vi "SUB instantant_frequency.vi"(2 "trimmed percent":cluster{"upper":dbl, "lower":dbl} {"lower" min=0.0 max=100.0 format="%#_g %"; "upper" min=0.0 max=100.0 format="%#_g %"}, 3 "scale info":variant, 4 "Omega":cluster{"frequency":dbl, "+- f":dbl}={"frequency"=444.0, "+- f"=50.0}, 5 "scalogram matrix":dbl[][](array[numeric])) -> (0 "IBandwidth":waveform(dbl), 1 "InstFrequency":waveform(dbl))   [LabVIEW 2017]
uses:
  <vilib>/addons/_Advanced Signal Processing/NI_AdvSigProcTFA.lvlib
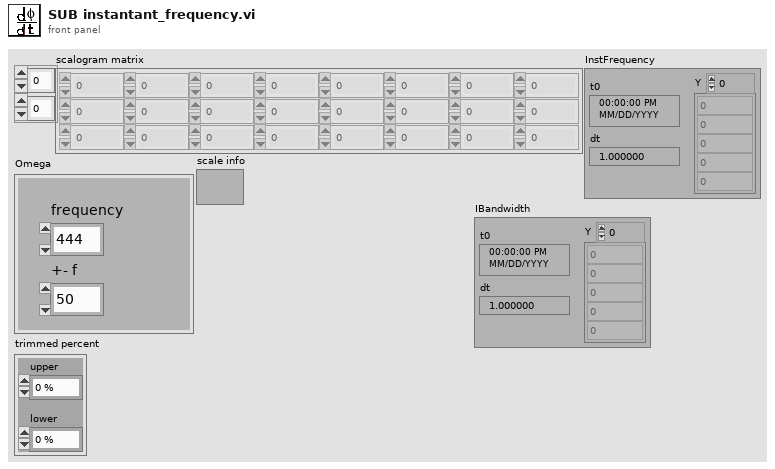
[diagram p1: front panel]
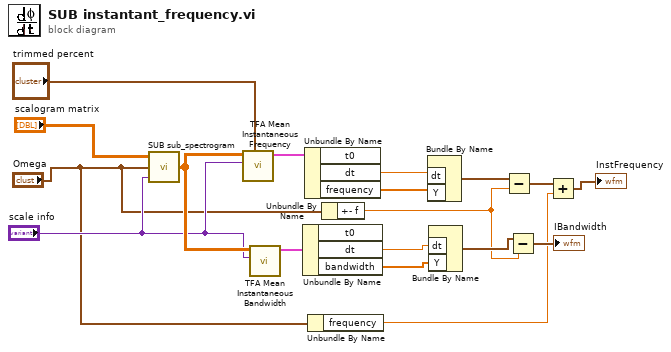
[diagram p0: block diagram]
diagram:
  n1 = call "SUB sub_spectrogram.vi"("scale info"="scale info", "Bandwidth"="Omega", "scalogram matrix"="scalogram matrix") -> ("sub_Spectrogram"=w14:cdb[][])
  n2 = call <vilib>:"TFA Mean Instantaneous Frequency.vi"("trimmed percent"="trimmed percent", "scale info"="scale info", "spectrogram"=w14) -> ("MIF"=w18:cluster{"t0":dbl, "dt":dbl, "frequency":dbl[]})  [unwired: 7 in, 1 out]
  n3 = call <vilib>:"TFA Mean Instantaneous Bandwidth.vi"("scale info"="scale info", "spectrogram"=w14) -> ("MIB"=w12:cluster{"t0":dbl, "dt":dbl, "bandwidth":dbl[]})  [unwired: 8 in, 1 out]
  n4 = Unbundle By Name(w12) -> ("dt"=w10:dbl, "bandwidth"=w9:dbl[])  [unwired: 1 out]
  n5 = Unbundle By Name(w18) -> ("dt"=w17:dbl, "frequency"=w16:dbl[])  [unwired: 1 out]
  n6 = Unbundle By Name("Omega") -> ("frequency"=w1:dbl)
  n7 = Unbundle By Name("Omega") -> ("+- f"=w7:dbl)
  n8 = Bundle By Name("dt"=w17, "Y"=w16) -> (w11:waveform(dbl))  [unwired: 1 in]
  n9 = Bundle By Name("dt"=w10, "Y"=w9) -> (w8:waveform(dbl))  [unwired: 1 in]
  n10 = Subtract(x=w11, y=w7) -> (x-y=w3:waveform(dbl))
  n11 = Subtract(x=w8, y=w7) -> (x-y=→"IBandwidth":waveform(dbl))
  n12 = Add(x=w3, y=w1) -> (x+y=→"InstFrequency":waveform(dbl))
